vi "table_sort.vi"(10 "Table in":string[][](array[string])=[["531421606102024020006A1105000100", "10/6/2024 4:31:53 PM", "C", "0.55", "OK", "", "", "", "", "", "", "", "", "", "", "", "", "", "", "", "", "", "", "", "", "", "", "", "", "", "", "", "", "", "", "", "", "", "", "", "", "", "", "", "", "", "", "", "", "", "", "", "", "", "", "", "", "", "", "", "", "", "", "", "", "", "", "", "", "", "", "", "", "", "", "", "", ""], ["531421606102024020007A1105000100", "10/6/2024 4:32:35 PM", "C", "0.51", "OK", "", "", "", "", "", "", "", "", "", "", "", "", "", "", "", "", "", "", "", "", "", "", "", "", "", "", "", "", "", "", "", "", "", "", "", "", "", "", "", "", "", "", "", "", "", "", "", "", "", "", "", "", "", "", "", "", "", "", "", "", "", "", "", "", "", "", "", "", "", "", "", "", ""], ["531421606102024020008A1105000100", "10/6/2024 4:33:15 PM", "C", "0.49", "OK", "", "", "", "", "", "", "", "", "", "", "", "", "", "", "", "", "", "", "", "", "", "", "", "", "", "", "", "", "", "", "", "", "", "", "", "", "", "", "", "", "", "", "", "", "", "", "", "", "", "", "", "", "", "", "", "", "", "", "", "", "", "", "", "", "", "", "", "", "", "", "", "", ""], ["531421606102024020009A1105000100", "10/6/2024 4:34:40 PM", "C", "0.54", "OK", "", "", "", "", "", "", "", "", "", "", "", "", "", "", "", "", "", "", "", "", "", "", "", "", "", "", "", "", "", "", "", "", "", "", "", "", "", "", "", "", "", "", "", "", "", "", "", "", "", "", "", "", "", "", "", "", "", "", "", "", "", "", "", "", "", "", "", "", "", "", "", "", ""], ["531421606102024020010A1105000100", "10/6/2024 4:35:18 PM", "C", "0.49", "OK", "", "", "", "", "", "", "", "", "", "", "", "", "", "", "", "", "", "", "", "", "", "", "", "", "", "", "", "", "", "", "", "", "", "", "", "", "", "", "", "", "", "", "", "", "", "", "", "", "", "", "", "", "", "", "", "", "", "", "", "", "", "", "", "", "", "", "", "", "", "", "", "", ""], ["531421606102024020011A1105000100", "10/6/2024 5:14:26 PM", "C", "0.56", "OK", "", "", "", "", "", "", "", "", "", "", "", "", "", "", "", "", "", "", "", "", "", "", "", "", "", "", "", "", "", "", "", "", "", "", "", "", "", "", "", "", "", "", "", "", "", "", "", "", "", "", "", "", "", "", "", "", "", "", "", "", "", "", "", "", "", "", "", "", "", "", "", "", ""], ["531421607102024020003A1105000100", "10/7/2024 3:29:30 PM", "B", "0.51", "OK", "", "", "", "", "", "", "", "", "", "", "", "", "", "", "", "", "", "", "", "", "", "", "", "", "", "", "", "", "", "", "", "", "", "", "", "", "", "", "", "", "", "", "", "", "", "", "", "", "", "", "", "", "", "", "", "", "", "", "", "", "", "", "", "", "", "", "", "", "", "", "", "", ""], ["531421607102024020004A1105000100", "10/7/2024 5:24:43 PM", "B", "0.37", "OK", "", "", "", "", "", "", "", "", "", "", "", "", "", "", "", "", "", "", "", "", "", "", "", "", "", "", "", "", "", "", "", "", "", "", "", "", "", "", "", "", "", "", "", "", "", "", "", "", "", "", "", "", "", "", "", "", "", "", "", "", "", "", "", "", "", "", "", "", "", "", "", "", ""], ["612413507102024020005A1105000100", "10/7/2024 5:42:21 PM", "B", "0.54", "OK", "", "", "", "", "", "", "", "", "", "", "", "", "", "", "", "", "", "", "", "", "", "", "", "", "", "", "", "", "", "", "", "", "", "", "", "", "", "", "", "", "", "", "", "", "", "", "", "", "", "", "", "", "", "", "", "", "", "", "", "", "", "", "", "", "", "", "", "", "", "", "", "", ""], ["612413507102024020006A1105000100", "10/7/2024 6:07:36 PM", "B", "0.52", "OK", "", "", "", "", "", "", "", "", "", "", "", "", "", "", "", "", "", "", "", "", "", "", "", "", "", "", "", "", "", "", "", "", "", "", "", "", "", "", "", "", "", "", "", "", "", "", "", "", "", "", "", "", "", "", "", "", "", "", "", "", "", "", "", "", "", "", "", "", "", "", "", "", ""], ["612413507102024020008A1105000100", "10/7/2024 6:19:01 PM", "B", "1.71", "OK", "", "", "", "", "", "", "", "", "", "", "", "", "", "", "", "", "", "", "", "", "", "", "", "", "", "", "", "", "", "", "", "", "", "", "", "", "", "", "", "", "", "", "", "", "", "", "", "", "", "", "", "", "", "", "", "", "", "", "", "", "", "", "", "", "", "", "", "", "", "", "", "", ""], ["612413507102024020009A1105000100", "10/7/2024 6:22:25 PM", "B", "0.54", "OK", "", "", "", "", "", "", "", "", "", "", "", "", "", "", "", "", "", "", "", "", "", "", "", "", "", "", "", "", "", "", "", "", "", "", "", "", "", "", "", "", "", "", "", "", "", "", "", "", "", "", "", "", "", "", "", "", "", "", "", "", "", "", "", "", "", "", "", "", "", "", "", "", ""], ["612413507102024020010A1105000100", "10/7/2024 6:23:51 PM", "B", "0.49", "OK", "", "", "", "", "", "", "", "", "", "", "", "", "", "", "", "", "", "", "", "", "", "", "", "", "", "", "", "", "", "", "", "", "", "", "", "", "", "", "", "", "", "", "", "", "", "", "", "", "", "", "", "", "", "", "", "", "", "", "", "", "", "", "", "", "", "", "", "", "", "", "", "", ""], ["612413507102024020011A1105000100", "10/7/2024 6:24:56 PM", "B", "0.51", "OK", "", "", "", "", "", "", "", "", "", "", "", "", "", "", "", "", "", "", "", "", "", "", "", "", "", "", "", "", "", "", "", "", "", "", "", "", "", "", "", "", "", "", "", "", "", "", "", "", "", "", "", "", "", "", "", "", "", "", "", "", "", "", "", "", "", "", "", "", "", "", "", "", ""], ["612413507102024020012A1105000100", "10/7/2024 7:00:38 PM", "B", "0.55", "OK", "", "", "", "", "", "", "", "", "", "", "", "", "", "", "", "", "", "", "", "", "", "", "", "", "", "", "", "", "", "", "", "", "", "", "", "", "", "", "", "", "", "", "", "", "", "", "", "", "", "", "", "", "", "", "", "", "", "", "", "", "", "", "", "", "", "", "", "", "", "", "", "", ""], ["612413507102024020013A1105000100", "10/7/2024 8:14:48 PM", "B", "0.56", "OK", "", "", "", "", "", "", "", "", "", "", "", "", "", "", "", "", "", "", "", "", "", "", "", "", "", "", "", "", "", "", "", "", "", "", "", "", "", "", "", "", "", "", "", "", "", "", "", "", "", "", "", "", "", "", "", "", "", "", "", "", "", "", "", "", "", "", "", "", "", "", "", "", ""], ["6124135", "10/7/2024 8:14:48 PM", "A", "", "", "", "", "", "", "", "", "", "", "", "", "", "", "", "", "", "", "", "", "", "", "", "", "", "", "", "", "", "", "", "", "", "", "", "", "", "", "", "", "", "", "", "", "", "", "", "", "", "", "", "", "", "", "", "", "", "", "", "", "", "", "", "", "", "", "", "", "", "", "", "", "", "", ""], ["07102024020013", "10/7/2024 8:14:48 PM", "A", "", "", "", "", "", "", "", "", "", "", "", "", "", "", "", "", "", "", "", "", "", "", "", "", "", "", "", "", "", "", "", "", "", "", "", "", "", "", "", "", "", "", "", "", "", "", "", "", "", "", "", "", "", "", "", "", "", "", "", "", "", "", "", "", "", "", "", "", "", "", "", "", "", "", ""], ["A1105000100", "10/7/2024 8:14:48 PM", "B", "0.56", "OK", "", "", "", "", "", "", "", "", "", "", "", "", "", "", "", "", "", "", "", "", "", "", "", "", "", "", "", "", "", "", "", "", "", "", "", "", "", "", "", "", "", "", "", "", "", "", "", "", "", "", "", "", "", "", "", "", "", "", "", "", "", "", "", "", "", "", "", "", "", "", "", "", ""], ["A1105000100", "10/8/2024 8:14:48 PM", "B", "0.56", "OK", "", "", "", "", "", "", "", "", "", "", "", "", "", "", "", "", "", "", "", "", "", "", "", "", "", "", "", "", "", "", "", "", "", "", "", "", "", "", "", "", "", "", "", "", "", "", "", "", "", "", "", "", "", "", "", "", "", "", "", "", "", "", "", "", "", "", "", "", "", "", "", "", ""], ["A1105000100", "10/8/2024 8:14:58 PM", "B", "0.56", "OK", "", "", "", "", "", "", "", "", "", "", "", "", "", "", "", "", "", "", "", "", "", "", "", "", "", "", "", "", "", "", "", "", "", "", "", "", "", "", "", "", "", "", "", "", "", "", "", "", "", "", "", "", "", "", "", "", "", "", "", "", "", "", "", "", "", "", "", "", "", "", "", "", ""]]) -> (3 "Table":string[][](array[string]))   [LabVIEW 2017]
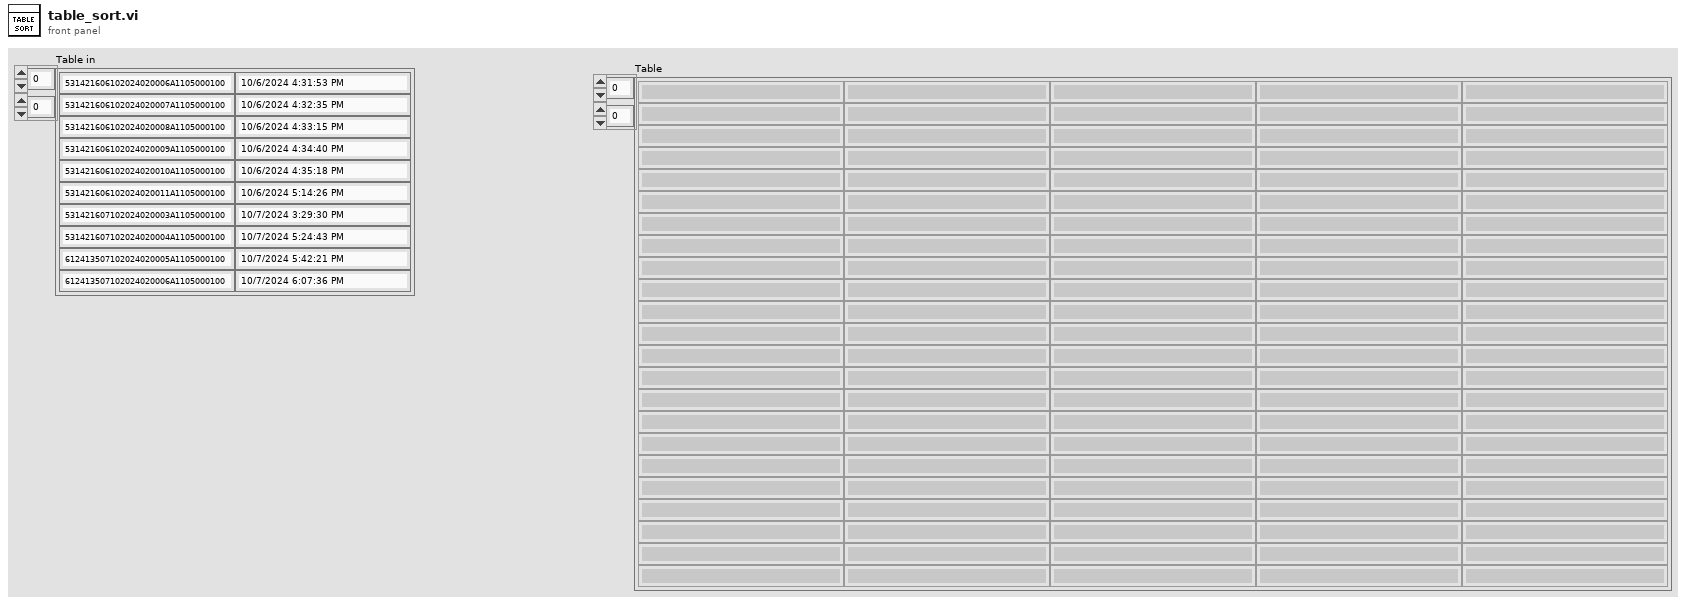
[diagram p1: front panel]
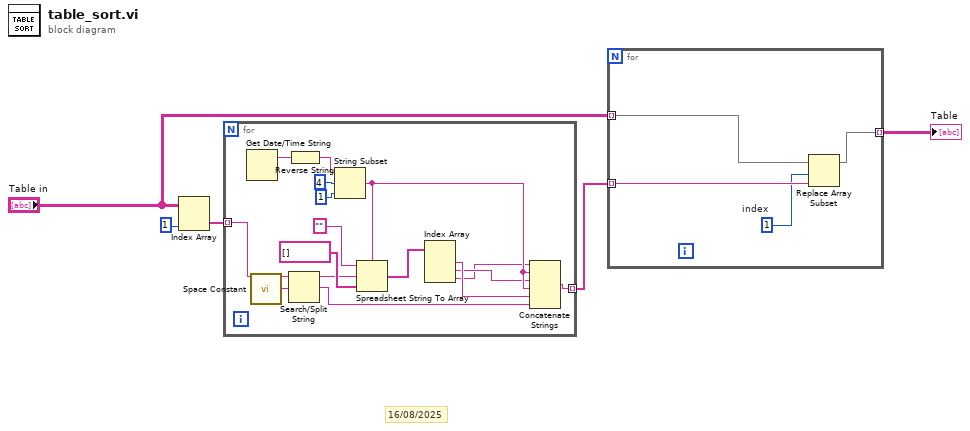
[diagram p0: block diagram]
diagram:
  # "16/08/2025"
  n1 = Index Array(array="Table in", index (col)=1 ("disabled index (col)")) -> (element=w4:string[])  [unwired: 1 in]
  n2 = for {
    tunnel: w4 -> [w21] mode=indexing
    tunnel: [w9] -> w3 mode=indexing
    n3 = Get Date/Time String() -> (date string=w18:string)  [unwired: 3 in, 1 out]
    n4 = call <vilib>:"Space Constant.vi"() -> ("String"=w16:string)
    n5 = Search/Split String(string=w21, search string/char (-)=w16) -> (substring before match=w14:string, match + rest of string=w10:string)  [unwired: 1 in, 1 out]
    n6 = Reverse String(1:w18) -> (0:w17:string)
    n7 = String Subset(string=w17, offset (0)=4, length (rest)=1 ("length (rest)")) -> (substring=w11:string)
    n8 = Spreadsheet String To Array(delimiter (Tab)=w11, format string="" ("String"), spreadsheet string=w14, array type (2D Dbl)=string[] []) -> (array=w12:string[])
    n9 = Index Array(array=w12) -> (element #1=w8:string, element #2=w7:string, element #3=w6:string)  [unwired: 3 in]
    n10 = Concatenate Strings(w6, w11, w7, w11, w8, w10) -> (w9:string)
  }
  n11 = for {
    tunnel: "Table in" -> [w23] mode=indexing
    tunnel: [w25] -> w1 mode=indexing
    tunnel: w3 -> [w24] mode=indexing
    w22 = 1  # index
    n12 = Replace Array Subset(array=w23, new element=w24, index=w22) -> (w25:string[])
  }
  "Table" <- w1
